vi "saveImageData.vi"(8 "error in":errorcluster, 9 "Robot Position 2":i32, 10 "data path":path, 11 "temp path":path) -> (0 "error out":errorcluster)   [LabVIEW 2012]
uses:
  <vilib>/Platform/TimedLoop/XDataNode/timing_clust.ctl
  <vilib>/Platform/TimedLoop/XDataNode/nitl_modes.ctl
  <vilib>/Platform/TimedLoop/XDataNode/wakeup.ctl
  GlobalBaslerCamera.vi
  <vilib>/Platform/TimedLoop/XDataNode/XDataNode.xnode
  <vilib>/Platform/TimedLoop/XDataNode/XDNodeRunTimeDep.lvlib
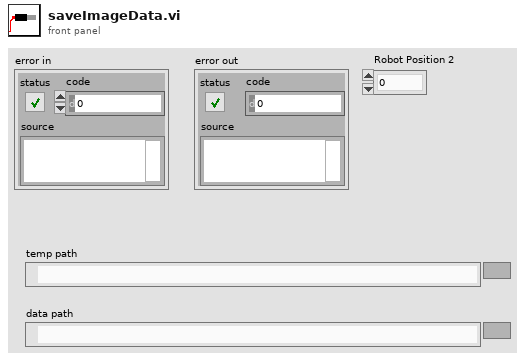
[diagram p1: front panel]
types:
  T1 = enum16{"open", "replace", "create", "open or create", "replace or create", "replace or create with confirmation"}
  T2 = typedef "XDNodeRunTimeDep.lvlib/timing_clust.ctl" = cluster{"Expected End [f-1]":u64, "Actual End [f-1]":u64, "Finished Late? [f-1]":bool, "Expected End [i-1]":u64, "Actual End [i-1]":u64, "Finished Late? [i-1]":bool, "Expected Start [i]":u64, "Actual Start [i]":u64, "Expected Start [f]":u64, "Actual Start [f]":u64, "Source Name":string, "Structure Name":string, "Period":i64, "Deadline":i64, "Offset":i64, "Start":i64, "Priority":i32, "Timeout":i32, "Mode":T3, "Wakeup Reason":T4, "Error":errorcluster, "Source Type":string, "Secondary Source Type":string, "Global End Time":u64, "Global Start Time":u64, "Frame Duration":u64, "Iteration Duration":u64, "Assigned CPU":i32, "I/O Scan Engine Mode":u32}
  T3 = typedef "XDNodeRunTimeDep.lvlib/nitl_modes.ctl" = enum32{"No Change", "Process missed periods, maintain original phase", "Discard missed periods, maintain original phase", "Process missed periods, ignore original phase", "Discard missed periods, ignore original phase"}
  T4 = typedef "XDNodeRunTimeDep.lvlib/wakeup.ctl" = enum32{"Normal", "Aborted", "Asynchronous wakeup", "Timing source error", "Timed loop error", "Timeout"}
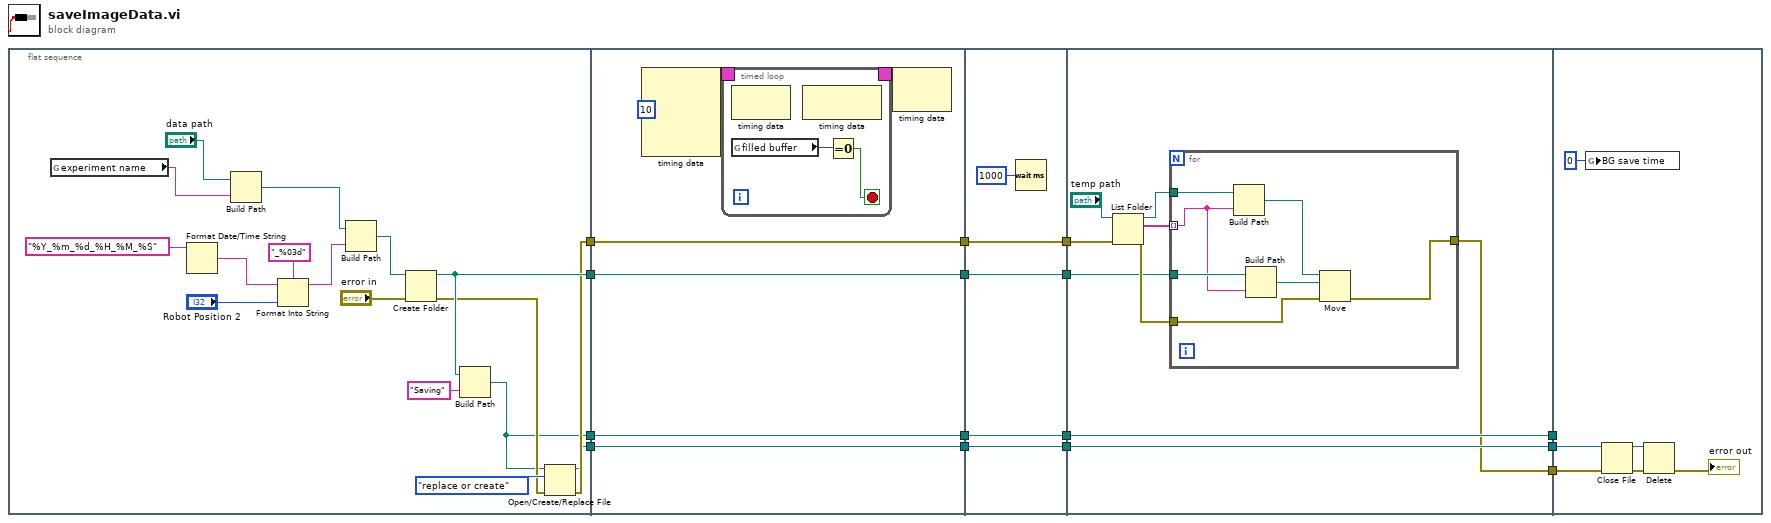
[diagram p0: block diagram]
diagram:
  n1 = flat-sequence {
    tunnel: [w21] -> w15
    tunnel: [w18] -> w14
    tunnel: [w17] -> w6
    tunnel: [w16] -> w2
    tunnel: w15 -> [w39]
    tunnel: [w39] -> w13
    tunnel: w14 -> [w38]
    tunnel: [w38] -> w11
    tunnel: [w34] -> w7
    tunnel: w6 -> [w34]
    tunnel: [w33] -> w3
    tunnel: w2 -> [w33]
    tunnel: w13 -> [w52]
    tunnel: [w52] -> w12
    tunnel: w11 -> [w51]
    tunnel: [w51] -> w10
    tunnel: [w49] -> w8
    tunnel: w7 -> [w49]
    tunnel: [w48] -> w4
    tunnel: w3 -> [w48]
    tunnel: w12 -> [w57]
    tunnel: w10 -> [w56]
    tunnel: [w55] -> w9
    tunnel: w8 -> [w55]
    tunnel: [w54] -> w5
    tunnel: w4 -> [w54]
    tunnel: [w53] -> w1
    tunnel: w9 -> [_]
    tunnel: w5 -> [w73]
    tunnel: w1 -> [w72]
    frame #0 {
      n2 = global read "GlobalBaslerCamera.vi" "experiment name"() -> (w25:string)
      n3 = Format Date/Time String(time format string (%c)="%Y_%m_%d_%H_%M_%S") -> (date/time string=w30:string)  [unwired: 2 in]
      n4 = Build Path(base path="data path", name or relative path=w25) -> (appended path=w23:path)
      n5 = Format Into String(format string="_%03d", initial string=w30, "Robot Position 2") -> (resulting string=w28:string)  [unwired: 1 in, 1 out]
      n6 = Build Path(base path=w23, name or relative path=w28) -> (appended path=w26:path)
      n7 = Create Folder(path (use dialog)=w26, error in="error in") -> (created path=w21:path, error out=w19:errorcluster)  [unwired: 1 in, 1 out]
      n8 = Build Path(base path=w21, name or relative path="Saving") -> (appended path=w17:path)
      n9 = Open/Create/Replace File(file path (use dialog)=w17, error in=w19, operation (0:open)=T1."replace or create") -> (refnum out=w16:refnum<file>, error out=w18:errorcluster)  [unwired: 3 in, 1 out]
    }
    frame #1 {
      n10 = node-c288(i64 10 ("Period")) -> (w37:T2)  [unwired: 3 in]
      n11 = timed-loop {
        timing: w37 -> [_]
        timing-out: [_] -> w36
        stop <- w40 stop-if-true
        n12 = node-c288() -> ()  [unwired: 1 in, 1 out]
        n13 = global read "GlobalBaslerCamera.vi" "filled buffer"() -> (w41:i32)
        n14 = node-c288() -> ()  [unwired: 1 in, 1 out]
        n15 = Equal To 0?(x=w41) -> (x = 0?=w40:bool)
      }
      n16 = node-c288(w36) -> ()  [unwired: 1 out]
    }
    frame #2 {
      n17 = Wait (ms)(milliseconds to wait=u32 1000) -> ()  [unwired: 1 out]
    }
    frame #3 {
      n18 = List Folder(path="temp path", error in=w56) -> (path out=w60:path, filenames=w59:string[], error out=w61:errorcluster)  [unwired: 2 in, 1 out]
      n19 = for {
        tunnel: w59 -> [w65] mode=indexing
        tunnel: w60 -> [w68]
        tunnel: w61 -> [w63]
        tunnel: [w62] -> w53
        tunnel: w57 -> [w66]
        n20 = Build Path(base path=w68, name or relative path=w65) -> (appended path=w67:path)
        n21 = Build Path(base path=w66, name or relative path=w65) -> (appended path=w64:path)
        n22 = Move(source path=w67, error in=w63, 10:w64) -> (error out=w62:errorcluster)  [unwired: 2 in, 2 out]
      }
    }
    frame #4 {
      n23 = global write "GlobalBaslerCamera.vi" "BG save time"(u32 0 ("BG save time")) -> ()
      n24 = Close File(refnum=w73, error in=w72) -> (path=w70:path, error out=w71:errorcluster)
      n25 = Delete(path (use dialog)=w70, error in=w71) -> (error out=→"error out":errorcluster)  [unwired: 3 in, 2 out]
    }
  }
